vi "Send Engine Pointer to Async Threads.vi"(8 "error in (no error)":errorcluster, 11 "Framework in":refnum<class "Framework.lvclass">) -> (0 "error out":errorcluster, 3 "Framework out":refnum<class "Framework.lvclass">)   [LabVIEW 2017, in "Data Sharing Framework Core.lvlib" / "Data Sharing Framework Engine.lvlib" / "Framework.lvclass"]
uses:
  Framework.lvclass
  Framework.lvclass/Framework.ctl
  Plugin/Plugin.lvclass/Plugin.ctl
  Internal/Transceiver/Transceiver Thread/Transceiver Thread.lvclass
  Plugin/Plugin.lvclass
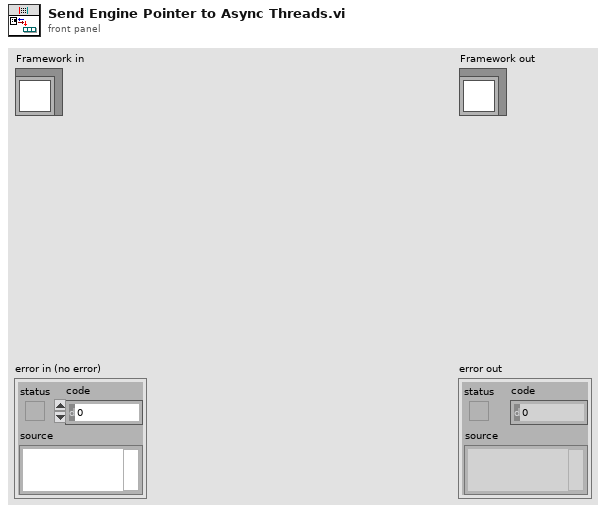
[diagram p1: front panel]
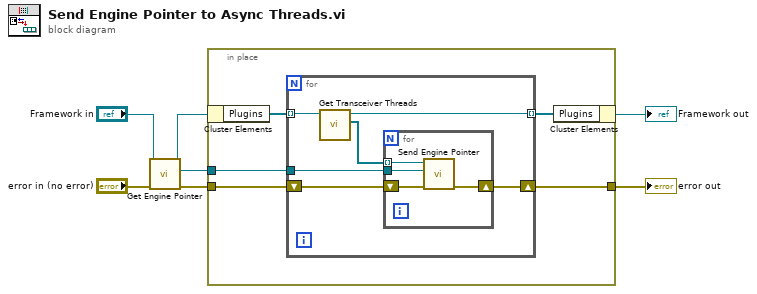
[diagram p0: block diagram]
diagram:
  n1 = call "Get Engine Pointer.vi"("Framework in"="Framework in") -> ("Engine Pointer"=w1:refnum<class "Memory.Pointer.lvclass">, "Framework out"=w2:refnum<class "Framework.lvclass">)  [unwired: 9 in]
  n2 = in-place {
    in-place-border: "error in (no error)" -> [w9]
    in-place-border: [w8] -> w4
    in-place-border: w1 -> [w7]
    n3 = in-place-cluster #1(w2) -> ("Plugins"=w11:refnum<class "Plugin.lvclass">[])
    n4 = for {
      tunnel: w11 -> [w17] mode=indexing
      tunnel: [w16] -> w10 mode=indexing
      shift-right: [w14] -> w8
      shift-left: w9 -> [w13]
      tunnel: w7 -> [w12]
      n5 = call "Get Transceiver Threads.vi"("Plugin in"=w17) -> ("Transceiver Threads"=w15:refnum<class "Transceiver Interface.lvclass">[], "Plugin out"=w16:refnum<class "Plugin.lvclass">)  [unwired: 9 in]
      n6 = for {
        tunnel: w15 -> [w21] mode=indexing
        shift-right: [w20] -> w14
        shift-left: w13 -> [w19]
        tunnel: w12 -> [w18]
        n7 = call "Send Engine Pointer.vi"("error in (no error)"=w19, "Engine Pointer"=w18, "Transceiver Interface in"=w21) -> ("error out"=w20:errorcluster)  [unwired: 7 in, 1 out]
      }
    }
    n8 = in-place-cluster #1("Plugins"=w10) -> (→"Framework out":refnum<class "Framework.lvclass">)
  }
  "error out" <- w4
